vi "main v1.2.vi"() -> ()   [LabVIEW 2015]
uses:
  <vilib>/userdefined/High Color/IMAQdx.ctl
  <vilib>/vision/driver/NI_Vision_Acquisition_Software.lvlib
panel:
  out "output variable":dbl
  out "XY Graph":cluster{dbl[], dbl[]}[](graph)
  out "Image Center Position:All Elements":cluster{"X":u32, "Y":u32}
  out "xc_green":dbl
  out "yc_green":dbl
  out "yc_red":dbl
  out "xc_red":dbl
  out "yc":dbl
  out "xc":dbl
  out "angle GREEN radian":dbl
  out "angle GREEN degree":dbl
  out "distance GREEN in cm":dbl
  out "angle RED radian":dbl
  out "angle RED degree":dbl
  out "distance RED in cm":dbl
  out "Original":T1(plugin-control)
  out "Green Landmark Detection":T1(plugin-control)
  in  "Green Landmark Position X":i32
  in  "Green Landmark Position Y":i32
  in  "Red Landmark Position Y":i32
  in  "Red Landmark Position X":i32
  out "Red ROI":T2
  out "Red Landmark Horizontal Side":i32
  out "Red Landmark Vertical Side":i32
  out "Red Landmark Center.Y":sgl
  out "Red Landmark Center.X":sgl
  out "Red Landmark Detection":T1(plugin-control)
  out "Number of Red Landmarks":i32
  out "Green ROI":T2
  out "Green Landmark Horizontal Side":i32
  out "Green Landmark Vertical Side":i32
  out "Green Landmark Center.Y":sgl
  out "Green Landmark Center.X":sgl
  out "Number of Green Landmarks":i32
  in  "stop":bool
  in  "Session In":T3
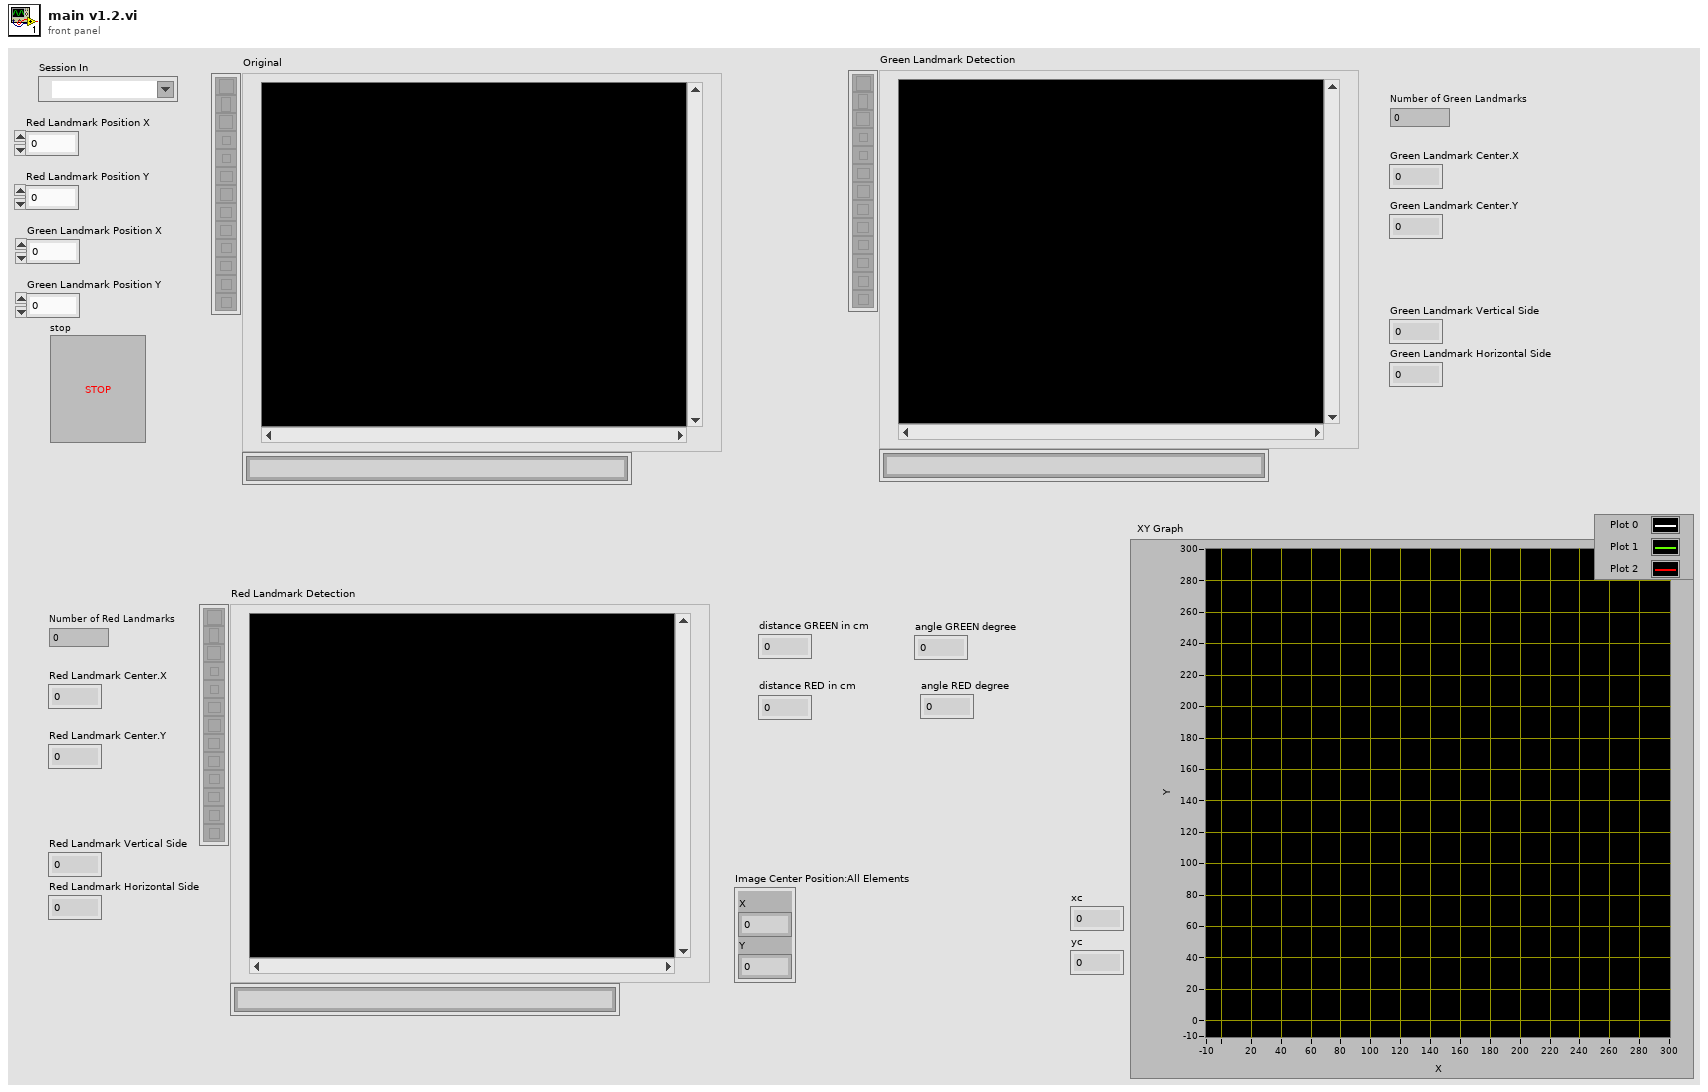
[diagram p1: front panel]
types:
  T1 = typedef "IMAQ Image.ctl" = refnum<image>
  T2 = cluster{"X Left":i32, "Y Top":i32, "X Right":i32, "Y Bottom":i32, "Rotation":i32}
  T3 = typedef "IMAQdx.ctl" = refnum<k21>
  T4 = typedef "Image Type" = u32
  T5 = enum16{"Landmark Detection", "ROI Landmark", "Red Landmark Distance calculation", "Green Landmark Distance calculation", "Camera Pose Estimation"}
  T6 = cluster{"Object Center":cluster{"X":sgl, "Y":sgl}, "Bounding Box":cluster{"X Left":i32, "Y Top":i32, "X Right":i32, "Y Bottom":i32}, "Area":sgl, "Orientation":sgl, "Aspect Ratio":sgl, "Nb Holes":i32}[]
  T7 = cluster{"Objects[0]":cluster{"Object Center":cluster{"X":sgl, "Y":sgl}, "Bounding Box":cluster{"X Left":i32, "Y Top":i32, "X Right":i32, "Y Bottom":i32}, "Area":sgl, "Orientation":sgl, "Aspect Ratio":sgl, "Nb Holes":i32}, "Objects[1]":cluster{"Object Center":cluster{"X":sgl, "Y":sgl}, "Bounding Box":cluster{"X Left":i32, "Y Top":i32, "X Right":i32, "Y Bottom":i32}, "Area":sgl, "Orientation":sgl, "Aspect Ratio":sgl, "Nb Holes":i32}, "Objects[2]":cluster{"Object Center":cluster{"X":sgl, "Y":sgl}, "Bounding Box":cluster{"X Left":i32, "Y Top":i32, "X Right":i32, "Y Bottom":i32}, "Area":sgl, "Orientation":sgl, "Aspect Ratio":sgl, "Nb Holes":i32}, "Objects[3]":cluster{"Object Center":cluster{"X":sgl, "Y":sgl}, "Bounding Box":cluster{"X Left":i32, "Y Top":i32, "X Right":i32, "Y Bottom":i32}, "Area":sgl, "Orientation":sgl, "Aspect Ratio":sgl, "Nb Holes":i32}, "Objects[4]":cluster{"Object Center":cluster{"X":sgl, "Y":sgl}, "Bounding Box":cluster{"X Left":i32, "Y Top":i32, "X Right":i32, "Y Bottom":i32}, "Area":sgl, "Orientation":sgl, "Aspect Ratio":sgl, "Nb Holes":i32}, "Objects[5]":cluster{"Object Center":cluster{"X":sgl, "Y":sgl}, "Bounding Box":cluster{"X Left":i32, "Y Top":i32, "X Right":i32, "Y Bottom":i32}, "Area":sgl, "Orientation":sgl, "Aspect Ratio":sgl, "Nb Holes":i32}, "Objects[6]":cluster{"Object Center":cluster{"X":sgl, "Y":sgl}, "Bounding Box":cluster{"X Left":i32, "Y Top":i32, "X Right":i32, "Y Bottom":i32}, "Area":sgl, "Orientation":sgl, "Aspect Ratio":sgl, "Nb Holes":i32}, "Objects[7]":cluster{"Object Center":cluster{"X":sgl, "Y":sgl}, "Bounding Box":cluster{"X Left":i32, "Y Top":i32, "X Right":i32, "Y Bottom":i32}, "Area":sgl, "Orientation":sgl, "Aspect Ratio":sgl, "Nb Holes":i32}, "Objects[8]":cluster{"Object Center":cluster{"X":sgl, "Y":sgl}, "Bounding Box":cluster{"X Left":i32, "Y Top":i32, "X Right":i32, "Y Bottom":i32}, "Area":sgl, "Orientation":sgl, "Aspect Ratio":sgl, "Nb Holes":i32}}
  T8 = cluster{"Object Center":cluster{"X":sgl, "Y":sgl}, "Bounding Box":cluster{"X Left":i32, "Y Top":i32, "X Right":i32, "Y Bottom":i32}, "Area":sgl, "Orientation":sgl, "Aspect Ratio":sgl, "Nb Holes":i32}
  T9 = cluster{"X Left":i32, "Y Top":i32, "X Right":i32, "Y Bottom":i32}
  T10 = typedef "ROI Descriptor" = cluster{"Global Rectangle":i32[], "Contours":cluster{"ID":enum32{"External", "Internal"}, "Type":u32, "Coordinates":i32[]}[]}
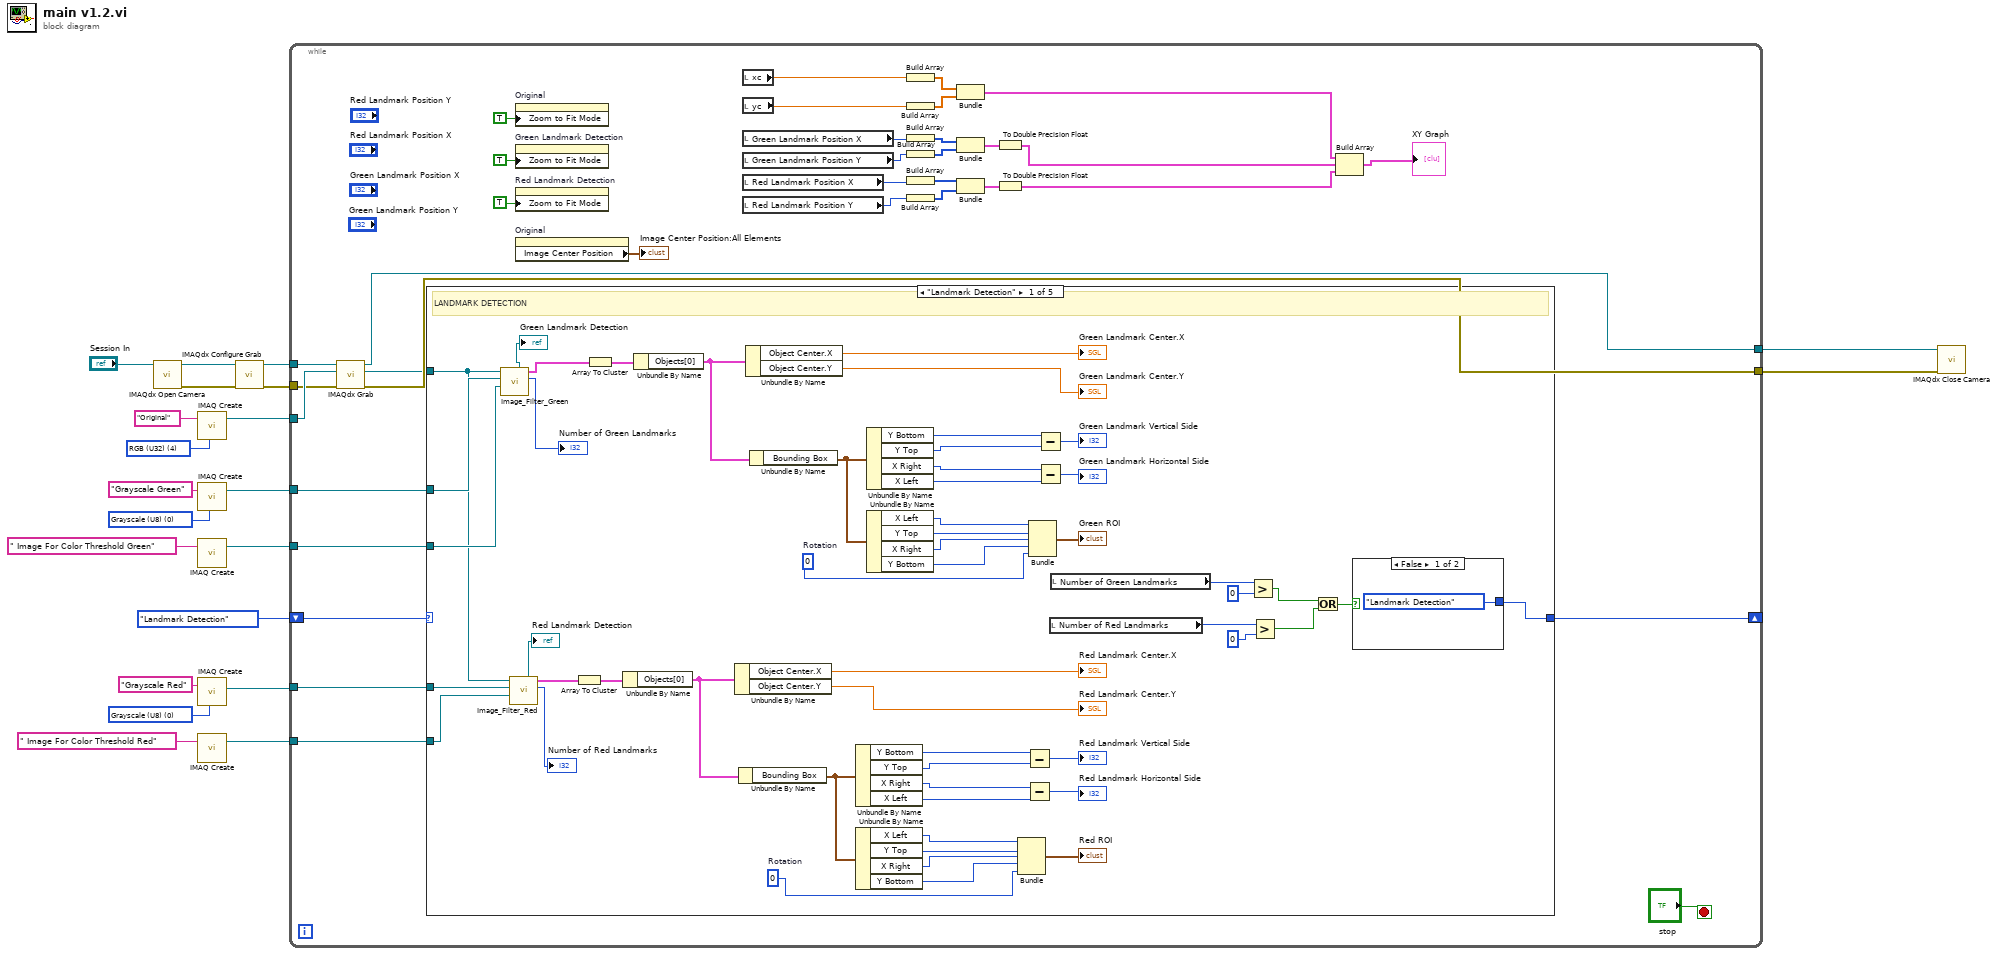
[diagram p0: block diagram]
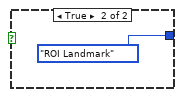
[diagram p2: hidden frame]
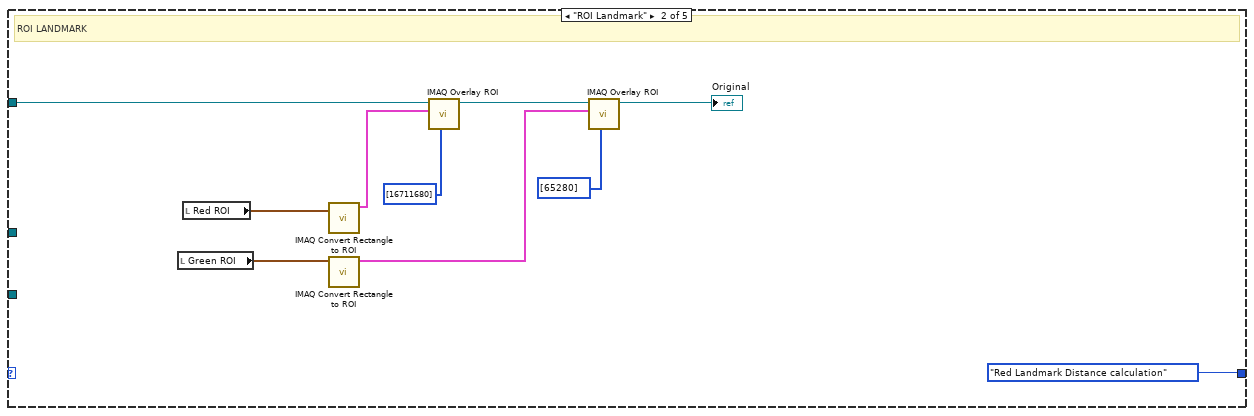
[diagram p3: hidden frame]
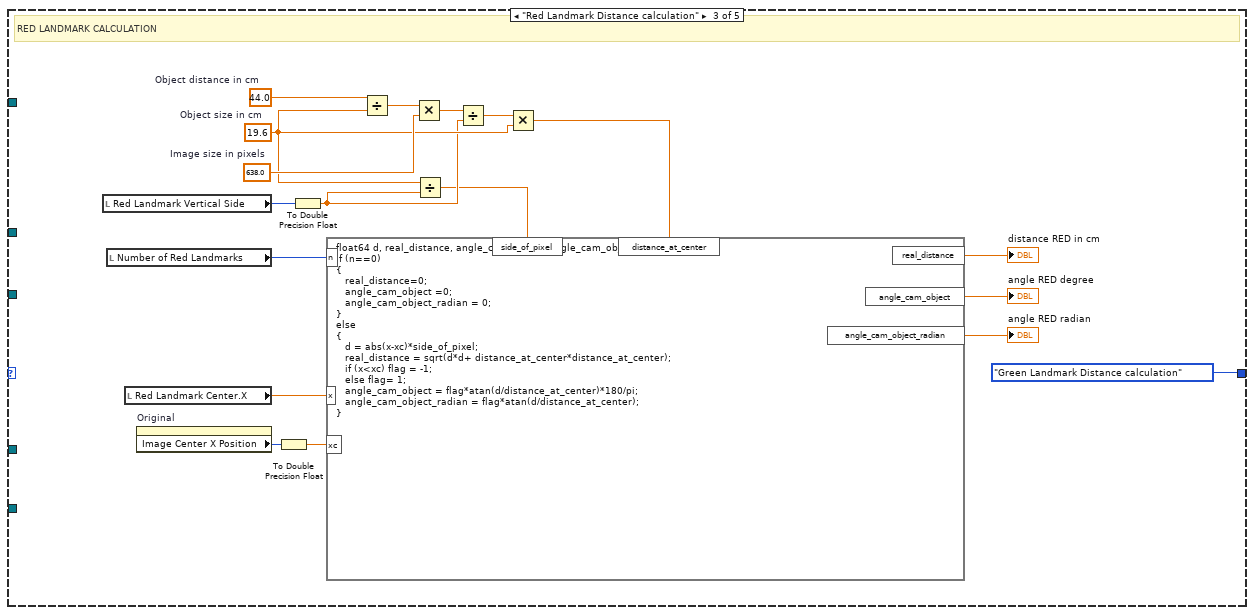
[diagram p4: hidden frame]
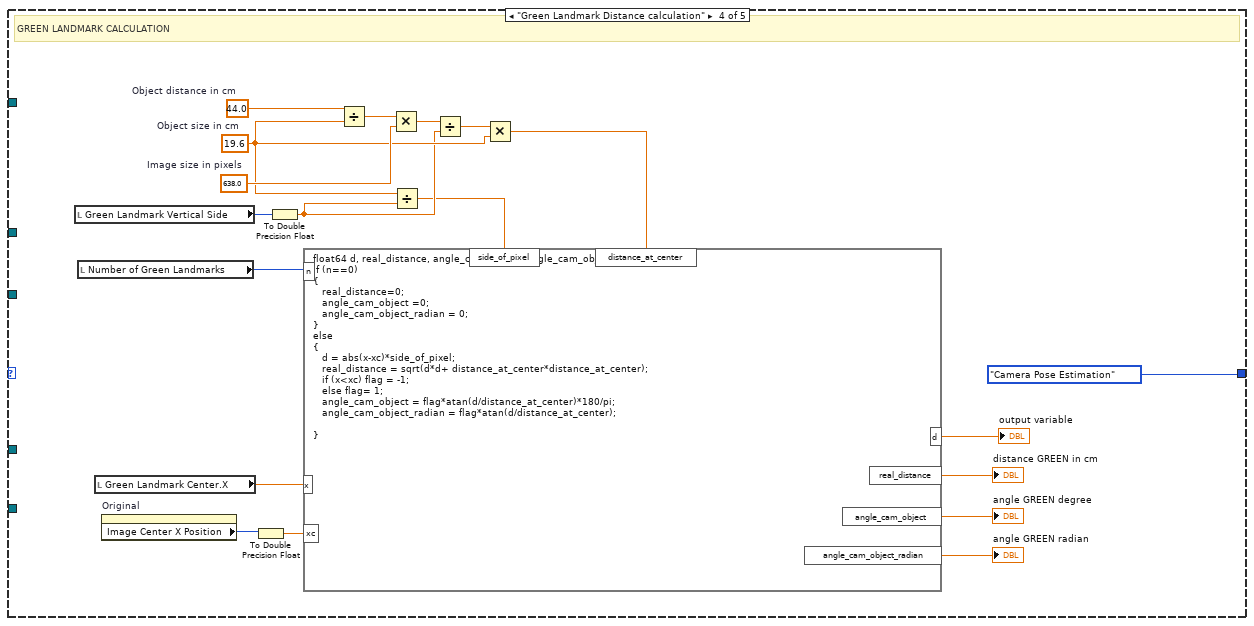
[diagram p5: hidden frame]
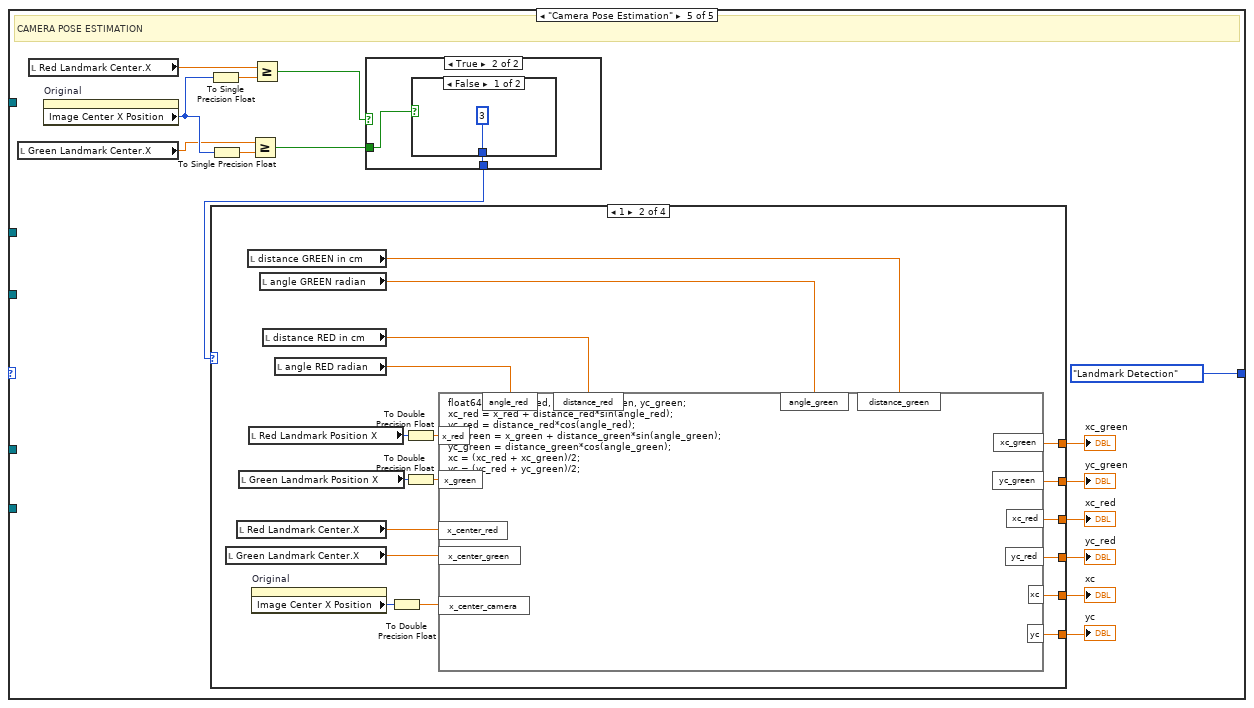
[diagram p6: hidden frame]
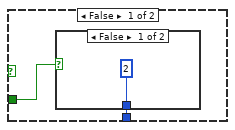
[diagram p7: hidden frame]
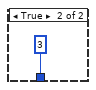
[diagram p8: hidden frame]
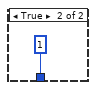
[diagram p9: hidden frame]
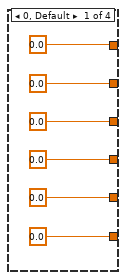
[diagram p10: hidden frame]
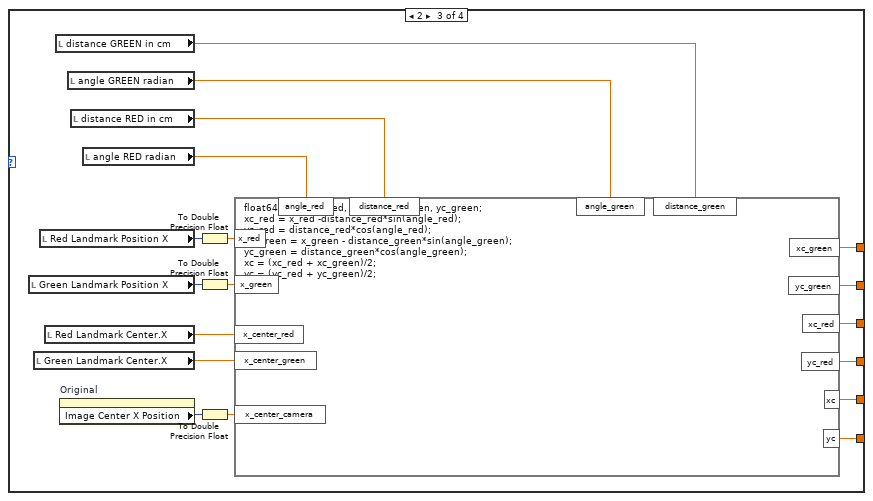
[diagram p11: hidden frame]
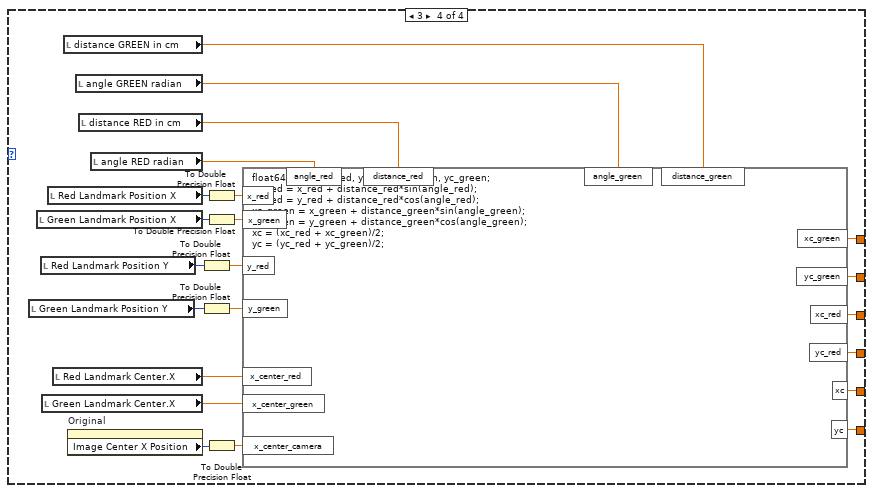
[diagram p12: hidden frame]
diagram:
  w4 = T4 0 items=["Grayscale (U8)", "Grayscale (I16)", "Grayscale (SGL)", "Complex (CSG)", "RGB (U32)", "HSL (U32)", "RGB (U64)", "Grayscale (U16)"] ("Image Type")
  w10 = T4 0 items=["Grayscale (U8)", "Grayscale (I16)", "Grayscale (SGL)", "Complex (CSG)", "RGB (U32)", "HSL (U32)", "RGB (U64)", "Grayscale (U16)"] ("Image Type")
  w14 = T4 4 items=["Grayscale (U8)", "Grayscale (I16)", "Grayscale (SGL)", "Complex (CSG)", "RGB (U32)", "HSL (U32)", "RGB (U64)", "Grayscale (U16)"] ("Image Type")
  n1 = call <vilib>:"IMAQdx Open Camera.vi"("Session In"="Session In") -> ("error out"=w18:errorcluster, "Session Out"=w21:T3)  [unwired: 9 in]
  n2 = call "IMAQ Create"("Image Name"="Original", "Image Type"=w14) -> ("New Image"=w17:T1)  [unwired: 3 in, 1 out]
  n3 = call "IMAQ Create"("Image Name"="Grayscale Green", "Image Type"=w10) -> ("New Image"=w8:T1)  [unwired: 3 in, 1 out]
  n4 = call "IMAQ Create"("Image Name"=" Image For Color Threshold Green") -> ("New Image"=w7:T1)  [unwired: 4 in, 1 out]
  n5 = call "IMAQ Create"("Image Name"="Grayscale Red", "Image Type"=w4) -> ("New Image"=w2:T1)  [unwired: 3 in, 1 out]
  n6 = call "IMAQ Create"("Image Name"=" Image For Color Threshold Red") -> ("New Image"=w1:T1)  [unwired: 4 in, 1 out]
  n7 = call <vilib>:"IMAQdx Configure Grab.vi"("error in"=w18, "Session In"=w21) -> ("error out"=w13:errorcluster, "Session Out"=w20:T3)  [unwired: 8 in]
  n8 = while {
    tunnel: w20 -> [w56]
    tunnel: w17 -> [w55]
    tunnel: [w49] -> w16
    tunnel: [w52] -> w15
    tunnel: w13 -> [w53]
    tunnel: w8 -> [w51]
    tunnel: w7 -> [w50]
    shift-right: [w44] -> _
    shift-left: T5."Landmark Detection" -> [w47]
    tunnel: w2 -> [w46]
    tunnel: w1 -> [w45]
    stop <- "stop" stop-if-true
    n9 = call <vilib>:"IMAQdx Grab.vi"("error in"=w53, "Image In"=w55, "Session In"=w56) -> ("error out"=w52:errorcluster, "Image Out"=w48:T1, "Session Out"=w49:T3)  [unwired: 5 in, 1 out]
    n10 = case shown="\"Landmark Detection\"" w47 {
      tunnel: w51 -> [w92 _ _ _ _]
      tunnel: w50 -> [w91 _ _ _ _]
      tunnel: w48 -> [w68 w119 _ _ _]
      tunnel: w46 -> [w67 _ _ _ _]
      tunnel: w45 -> [w66 _ _ _ _]
      tunnel: [w58 T5."Red Landmark Distance calculation" T5."Green Landmark Distance calculation" T5."Camera Pose Estimation" T5."Landmark Detection"] -> w44
      frame "Landmark Detection" {
        w70 = 0  # Rotation
        w94 = 0  # Rotation
        # "LANDMARK DETECTION"
        n11 = call "Image_Filter_Green.vi"("Input Image"=w68, "New Image of IMAQ Threshold"=w92, "New Image for Color Threshold"=w91) -> ("Output Image of Object Detection"=→"Green Landmark Detection":T1, "Objects"=w89:T6, "Number of Objects"=→"Number of Green Landmarks":i32)  [unwired: 4 in]
        n12 = call "Image_Filter_Red.vi"("Input Image"=w68, "New Image of IMAQ Threshold"=w67, "New Image for Color Threshold"=w66) -> ("Output Image of Object Detection"=→"Red Landmark Detection":T1, "Objects"=w86:T6, "Number of Objects"=→"Number of Red Landmarks":i32)  [unwired: 4 in]
        n13 = Array To Cluster(array=w86) -> (cluster=w85:T7)
        n14 = Array To Cluster(array=w89) -> (cluster=w109:T7)
        n15 = Unbundle By Name(w85) -> ("Objects[0]"=w84:T8)
        n16 = Unbundle By Name(w109) -> ("Objects[0]"=w108:T8)
        n17 = Unbundle By Name(w84) -> ("Object Center.X"=→"Red Landmark Center.X":sgl, "Object Center.Y"=→"Red Landmark Center.Y":sgl)
        n18 = Unbundle By Name(w84) -> ("Bounding Box"=w75:T9)
        n19 = Unbundle By Name(w108) -> ("Object Center.X"=→"Green Landmark Center.X":sgl, "Object Center.Y"=→"Green Landmark Center.Y":sgl)
        n20 = Unbundle By Name(w108) -> ("Bounding Box"=w99:T9)
        n21 = Unbundle By Name(w75) -> ("Y Bottom"=w81:i32, "Y Top"=w80:i32, "X Right"=w79:i32, "X Left"=w78:i32)
        n22 = Unbundle By Name(w75) -> ("X Left"=w74:i32, "Y Top"=w73:i32, "X Right"=w72:i32, "Y Bottom"=w71:i32)
        n23 = Unbundle By Name(w99) -> ("Y Bottom"=w105:i32, "Y Top"=w104:i32, "X Right"=w103:i32, "X Left"=w102:i32)
        n24 = Unbundle By Name(w99) -> ("X Left"=w98:i32, "Y Top"=w97:i32, "X Right"=w96:i32, "Y Bottom"=w95:i32)
        n25 = Bundle("X Left"=w74, "Y Top"=w73, "X Right"=w72, "Y Bottom"=w71, "Rotation"=w70) -> (→"Red ROI":T2)  [unwired: 1 in]
        n26 = Subtract(x=w81, y=w80) -> (x-y=→"Red Landmark Vertical Side":i32)
        n27 = Subtract(x=w79, y=w78) -> (x-y=→"Red Landmark Horizontal Side":i32)
        n28 = Bundle("X Left"=w98, "Y Top"=w97, "X Right"=w96, "Y Bottom"=w95, "Rotation"=w94) -> (→"Green ROI":T2)  [unwired: 1 in]
        n29 = Subtract(x=w105, y=w104) -> (x-y=→"Green Landmark Vertical Side":i32)
        n30 = Subtract(x=w103, y=w102) -> (x-y=→"Green Landmark Horizontal Side":i32)
        n31 = local read "Number of Red Landmarks"() -> (w63:i32)
        n32 = local read "Number of Green Landmarks"() -> (w65:i32)
        n33 = Greater?(x=w65, y=0) -> (0:w61:bool)
        n34 = Greater?(x=w63, y=0) -> (0:w60:bool)
        n35 = Or(x=w61, y=w60) -> (x .or. y?=w59:bool)
        n36 = case shown="False" w59 {
          tunnel: [T5."Landmark Detection" T5."ROI Landmark"] -> w58
          frame False {
          }
          frame True {
          }
        }
      }
      frame "ROI Landmark" {
        # "ROI LANDMARK"
        n37 = local read "Green ROI"() -> (w120:T2)
        n38 = local read "Red ROI"() -> (w121:T2)
        n39 = call "IMAQ Convert Rectangle to ROI"("Rectangle"=w121) -> ("ROI Descriptor"=w118:T10)  [unwired: 8 in, 1 out]
        n40 = call "IMAQ Convert Rectangle to ROI"("Rectangle"=w120) -> ("ROI Descriptor"=w115:T10)  [unwired: 8 in, 1 out]
        n41 = call "IMAQ Overlay ROI"("Colors (Green)"=u32[] [16711680], "ROI Descriptor"=w118, "Image"=w119) -> ("Image Out"=w116:T1)  [unwired: 7 in, 1 out]
        n42 = call "IMAQ Overlay ROI"("Colors (Green)"=u32[] [65280], "ROI Descriptor"=w115, "Image"=w116) -> ("Image Out"=→"Original":T1)  [unwired: 7 in, 1 out]
      }
      frame "Red Landmark Distance calculation" {
        w133 = 638.0  # Image size in pixels
        w132 = 19.6  # Object size in cm
        w137 = 44.0  # Object distance in cm
        # "RED LANDMARK CALCULATION"
        n43 = local read "Red Landmark Vertical Side"() -> (w138:i32)
        n44 = local read "Number of Red Landmarks"() -> (w122:i32)
        n45 = local read "Red Landmark Center.X"() -> (w130:sgl)
        n46 = property on="Original" class="ImageControl"() -> ("Image Center X Position"=w129:u32)  [unwired: 2 in, 2 out]
        n47 = To Double Precision Float(number=w129) -> (double precision float=w128:dbl)
        n48 = To Double Precision Float(number=w138) -> (double precision float=w131:dbl)
        n49 = Divide(x=w137, y=w132) -> (x/y=w136:dbl)
        n50 = Multiply(x=w136, y=w133) -> (x*y=w134:dbl)
        n51 = Divide(x=w132, y=w131) -> (x/y=w126:dbl)
        n52 = Divide(x=w134, y=w131) -> (x/y=w135:dbl)
        n53 = Multiply(x=w135, y=w132) -> (x*y=w127:dbl)
        n54 = formula code="float64 d, real_distance, angle_cam_object, angle_cam_object_radian,flag; \nif (n==0)\n{\n   real_distance=0;\n   angle_cam_object =0;\n   angle_cam_object_radian = 0;\n}\nelse\n{\n   d = abs(x-xc)*side_of_pixel;\n   real_distance = sqrt(d*d+ distance_at_center*distance_at_center);\n   if (x<xc) flag = -1;\n   else flag= 1;\n   angle_cam_object = flag*atan(d/distance_at_center)*180/pi;\n   angle_cam_object_radian = flag*atan(d/distance_at_center);\n}"("x"=w130, "xc"=w128, "distance_at_center"=w127, "side_of_pixel"=w126, "n"=w122) -> ("real_distance"=→"distance RED in cm":dbl, "angle_cam_object"=→"angle RED degree":dbl, "angle_cam_object_radian"=→"angle RED radian":dbl)
      }
      frame "Green Landmark Distance calculation" {
        w152 = 638.0  # Image size in pixels
        w151 = 19.6  # Object size in cm
        w156 = 44.0  # Object distance in cm
        # "GREEN LANDMARK CALCULATION"
        n55 = local read "Green Landmark Vertical Side"() -> (w157:i32)
        n56 = local read "Number of Green Landmarks"() -> (w141:i32)
        n57 = local read "Green Landmark Center.X"() -> (w149:sgl)
        n58 = property on="Original" class="ImageControl"() -> ("Image Center X Position"=w142:u32)  [unwired: 2 in, 2 out]
        n59 = To Double Precision Float(number=w142) -> (double precision float=w148:dbl)
        n60 = To Double Precision Float(number=w157) -> (double precision float=w150:dbl)
        n61 = Divide(x=w156, y=w151) -> (x/y=w155:dbl)
        n62 = Multiply(x=w155, y=w152) -> (x*y=w153:dbl)
        n63 = Divide(x=w151, y=w150) -> (x/y=w146:dbl)
        n64 = Divide(x=w153, y=w150) -> (x/y=w154:dbl)
        n65 = Multiply(x=w154, y=w151) -> (x*y=w147:dbl)
        n66 = formula code="float64 d, real_distance, angle_cam_object, angle_cam_object_radian, flag; \nif (n==0)\n{\n   real_distance=0;\n   angle_cam_object =0;\n   angle_cam_object_radian = 0;\n}\nelse\n{\n   d = abs(x-xc)*side_of_pixel;\n   real_distance = sqrt(d*d+ distance_at_center*distance_at_center);\n   if (x<xc) flag = -1;\n   else flag= 1;\n   angle_cam_object = flag*atan(d/distance_at_center)*180/pi;\n   angle_cam_object_radian = flag*atan(d/distance_at_center);\n\n}"("x"=w149, "xc"=w148, "distance_at_center"=w147, "side_of_pixel"=w146, "n"=w141) -> ("real_distance"=→"distance GREEN in cm":dbl, "angle_cam_object"=→"angle GREEN degree":dbl, "angle_cam_object_radian"=→"angle GREEN radian":dbl, "d"=→"output variable":dbl)
      }
      frame "Camera Pose Estimation" {
        # "CAMERA POSE ESTIMATION"
        n67 = local read "Green Landmark Center.X"() -> (w161:sgl)
        n68 = local read "Red Landmark Center.X"() -> (w166:sgl)
        n69 = property on="Original" class="ImageControl"() -> ("Image Center X Position"=w164:u32)  [unwired: 2 in, 2 out]
        n70 = To Single Precision Float(number=w164) -> (single precision float=w165:sgl)
        n71 = To Single Precision Float(number=w164) -> (single precision float=w160:sgl)
        n72 = Greater Or Equal?(x=w161, y=w160) -> (x >= y?=w159:bool)
        n73 = Greater Or Equal?(x=w166, y=w165) -> (x >= y?=w163:bool)
        n74 = case shown="True" w163 {
          tunnel: [w175 w179] -> w162
          tunnel: w159 -> [w174 w178]
          frame False {
            n75 = case shown="False" w174 {
              tunnel: [2 3] -> w175
              frame False {
              }
              frame True {
              }
            }
          }
          frame True {
            n76 = case shown="False" w178 {
              tunnel: [3 1] -> w179
              frame False {
              }
              frame True {
              }
            }
          }
        }
        n77 = case shown="1" w162 {
          tunnel: [0.0 w197 w219 w241] -> w172
          tunnel: [0.0 w196 w218 w240] -> w171
          tunnel: [0.0 w195 w221 w243] -> w170
          tunnel: [0.0 w194 w220 w242] -> w169
          tunnel: [0.0 w193 w222 w244] -> w168
          tunnel: [0.0 w192 w223 w245] -> w167
          frame 0, Default {
          }
          frame 1 {
            n78 = local read "Green Landmark Center.X"() -> (w204:sgl)
            n79 = local read "Red Landmark Center.X"() -> (w205:sgl)
            n80 = local read "Green Landmark Position X"() -> (w191:i32)
            n81 = local read "distance GREEN in cm"() -> (w199:dbl)
            n82 = local read "Red Landmark Position X"() -> (w189:i32)
            n83 = property on="Original" class="ImageControl"() -> ("Image Center X Position"=w202:u32)  [unwired: 2 in, 2 out]
            n84 = local read "angle GREEN radian"() -> (w198:dbl)
            n85 = local read "distance RED in cm"() -> (w200:dbl)
            n86 = local read "angle RED radian"() -> (w201:dbl)
            n87 = To Double Precision Float(number=w202) -> (double precision float=w203:dbl)
            n88 = To Double Precision Float(number=w189) -> (double precision float=w188:dbl)
            n89 = To Double Precision Float(number=w191) -> (double precision float=w190:dbl)
            n90 = formula code="float64 xc, yc, xc_red, yc_red, xc_green, yc_green;\nxc_red = x_red + distance_red*sin(angle_red);\nyc_red = distance_red*cos(angle_red);\nxc_green = x_green + distance_green*sin(angle_green);\nyc_green = distance_green*cos(angle_green);\nxc = (xc_red + xc_green)/2; \nyc = (yc_red + yc_green)/2;"("x_center_red"=w205, "x_center_green"=w204, "x_center_camera"=w203, "angle_red"=w201, "angle_green"=w198, "distance_red"=w200, "distance_green"=w199, "x_red"=w188, "x_green"=w190) -> ("xc"=w197:dbl, "yc"=w196:dbl, "xc_red"=w195:dbl, "yc_red"=w194:dbl, "xc_green"=w192:dbl, "yc_green"=w193:dbl)
          }
          frame 2 {
            n91 = local read "Green Landmark Position X"() -> (w211:i32)
            n92 = local read "Green Landmark Center.X"() -> (w206:sgl)
            n93 = local read "Red Landmark Position X"() -> (w208:i32)
            n94 = local read "Red Landmark Center.X"() -> (w207:sgl)
            n95 = local read "distance GREEN in cm"() -> (w214:dbl)
            n96 = property on="Original" class="ImageControl"() -> ("Image Center X Position"=w213:u32)  [unwired: 2 in, 2 out]
            n97 = local read "angle GREEN radian"() -> (w215:dbl)
            n98 = local read "distance RED in cm"() -> (w216:dbl)
            n99 = local read "angle RED radian"() -> (w217:dbl)
            n100 = To Double Precision Float(number=w208) -> (double precision float=w209:dbl)
            n101 = To Double Precision Float(number=w211) -> (double precision float=w210:dbl)
            n102 = To Double Precision Float(number=w213) -> (double precision float=w212:dbl)
            n103 = formula code="float64 xc, yc, xc_red, yc_red, xc_green, yc_green;\nxc_red = x_red -distance_red*sin(angle_red);\nyc_red = distance_red*cos(angle_red);\nxc_green = x_green - distance_green*sin(angle_green);\nyc_green = distance_green*cos(angle_green);\nxc = (xc_red + xc_green)/2; \nyc = (yc_red + yc_green)/2;"("x_center_red"=w207, "x_center_green"=w206, "x_center_camera"=w212, "angle_red"=w217, "angle_green"=w215, "distance_red"=w216, "distance_green"=w214, "x_red"=w209, "x_green"=w210) -> ("xc"=w219:dbl, "yc"=w218:dbl, "xc_red"=w221:dbl, "yc_red"=w220:dbl, "xc_green"=w223:dbl, "yc_green"=w222:dbl)
          }
          frame 3 {
            n104 = local read "Green Landmark Position Y"() -> (w225:i32)
            n105 = local read "Green Landmark Position X"() -> (w233:i32)
            n106 = local read "Red Landmark Position Y"() -> (w227:i32)
            n107 = local read "Green Landmark Center.X"() -> (w230:sgl)
            n108 = local read "Red Landmark Position X"() -> (w235:i32)
            n109 = local read "Red Landmark Center.X"() -> (w231:sgl)
            n110 = local read "distance GREEN in cm"() -> (w236:dbl)
            n111 = property on="Original" class="ImageControl"() -> ("Image Center X Position"=w229:u32)  [unwired: 2 in, 2 out]
            n112 = local read "angle GREEN radian"() -> (w237:dbl)
            n113 = local read "distance RED in cm"() -> (w238:dbl)
            n114 = local read "angle RED radian"() -> (w239:dbl)
            n115 = To Double Precision Float(number=w227) -> (double precision float=w226:dbl)
            n116 = To Double Precision Float(number=w225) -> (double precision float=w224:dbl)
            n117 = To Double Precision Float(number=w235) -> (double precision float=w234:dbl)
            n118 = To Double Precision Float(number=w233) -> (double precision float=w232:dbl)
            n119 = To Double Precision Float(number=w229) -> (double precision float=w228:dbl)
            n120 = formula code="float64 xc, yc, xc_red, yc_red, xc_green, yc_green;\nxc_red = x_red + distance_red*sin(angle_red);\nyc_red = y_red + distance_red*cos(angle_red);\nxc_green = x_green + distance_green*sin(angle_green);\nyc_green = y_green + distance_green*cos(angle_green);\nxc = (xc_red + xc_green)/2; \nyc = (yc_red + yc_green)/2;"("x_center_red"=w231, "x_center_green"=w230, "x_center_camera"=w228, "angle_red"=w239, "angle_green"=w237, "distance_red"=w238, "distance_green"=w236, "x_red"=w234, "x_green"=w232, "y_red"=w226, "y_green"=w224) -> ("xc"=w241:dbl, "yc"=w240:dbl, "xc_red"=w243:dbl, "yc_red"=w242:dbl, "xc_green"=w245:dbl, "yc_green"=w244:dbl)
          }
        }
        "xc" <- w172
        "yc" <- w171
        "xc_red" <- w170
        "yc_red" <- w169
        "yc_green" <- w168
        "xc_green" <- w167
      }
    }
    n121 = property on="Original" class="ImageControl"("Zoom to Fit Mode"=TRUE) -> ()  [unwired: 2 in, 2 out]
    n122 = property on="Green Landmark Detection" class="ImageControl"("Zoom to Fit Mode"=TRUE) -> ()  [unwired: 2 in, 2 out]
    n123 = property on="Red Landmark Detection" class="ImageControl"("Zoom to Fit Mode"=TRUE) -> ()  [unwired: 2 in, 2 out]
    n124 = property on="Original" class="ImageControl"() -> ("Image Center Position"=→"Image Center Position:All Elements":cluster{"X":u32, "Y":u32})  [unwired: 2 in, 2 out]
    n125 = local read "xc"() -> (w34:dbl)
    n126 = local read "yc"() -> (w32:dbl)
    n127 = local read "Green Landmark Position X"() -> (w30:i32)
    n128 = local read "Green Landmark Position Y"() -> (w28:i32)
    n129 = local read "Red Landmark Position X"() -> (w25:i32)
    n130 = local read "Red Landmark Position Y"() -> (w24:i32)
    n131 = Build Array(w34) -> (w33:dbl[])
    n132 = Build Array(w32) -> (w31:dbl[])
    n133 = Build Array(w30) -> (w29:i32[])
    n134 = Build Array(w28) -> (w27:i32[])
    n135 = Build Array(w25) -> (w26:i32[])
    n136 = Build Array(w24) -> (w23:i32[])
    n137 = Bundle(w33, w31) -> (w37:cluster{dbl[], dbl[]})  [unwired: 1 in]
    n138 = Bundle(w29, w27) -> (w39:cluster{i32[], i32[]})  [unwired: 1 in]
    n139 = Bundle(w26, w23) -> (w38:cluster{i32[], i32[]})  [unwired: 1 in]
    n140 = To Double Precision Float(number=w39) -> (double precision float=w35:cluster{dbl[], dbl[]})
    n141 = To Double Precision Float(number=w38) -> (double precision float=w36:cluster{dbl[], dbl[]})
    n142 = Build Array(w37, w35, w36) -> (→"XY Graph":cluster{dbl[], dbl[]}[])
  }
  n143 = call <vilib>:"IMAQdx Close Camera.vi"("error in"=w15, "Session In"=w16) -> ()  [unwired: 9 in, 1 out]
